vi "Get PPMS Class.vi"(8 "error in (no error)":errorcluster, 11 "instrument.PPMS":refnum<class "instrument.PPMS.lvclass">) -> (0 "error out":errorcluster, 2 "Select PPMS":T1, 3 "instrument.PPMS out":refnum<class "instrument.PPMS.lvclass">)   [LabVIEW 2019, in "PPMS.lvlib"]
uses:
  PPMS.lvlib
  Select PPMS--Enum.ctl
  instrument.PPMS/instrument.PPMS.lvclass
  instrument.PPMS1/instrument.PPMS1.lvclass
  C:/Users/patrick/Documents/GitHub/levylabpitt/PPMS-Monitor-and-Control/lvsrc/instrument.PPMS/instrument.PPMS.lvclass
  instrument.PPMS2/instrument.PPMS2.lvclass
  instrument.PPMS3/instrument.PPMS3.lvclass
  instrument.OptiCool/instrument.OptiCool.lvclass
  instrument.PPMS-W-1/instrument.PPMS-W-1.lvclass
  instrument.PPMS/instrument.PPMS.lvclass/instrument.PPMS.ctl
  C:/Program Files (x86)/National Instruments/LabVIEW 2019/user.lib/LevyLab/Instrument Framework/Instrument Types/Cryostat/Instrument.Cryostat.lvclass
  C:/Program Files (x86)/National Instruments/LabVIEW 2019/user.lib/LevyLab/Instrument Framework/Instrument/Instrument.lvclass
  C:/Program Files (x86)/National Instruments/LabVIEW 2019/vi.lib/JKI/JKI SMO/SMO/SMO.lvclass
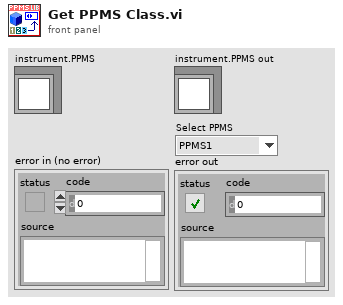
[diagram p1: front panel]
types:
  T1 = typedef "PPMS.lvlib/Select PPMS--Enum.ctl" = enum16{"PPMS1", "PPMS2", "PPMS3", "OptiCool", "PPMS-W-1", "Simulate PPMS", "Simulate DynaCool", "Simulate OptiCool"}
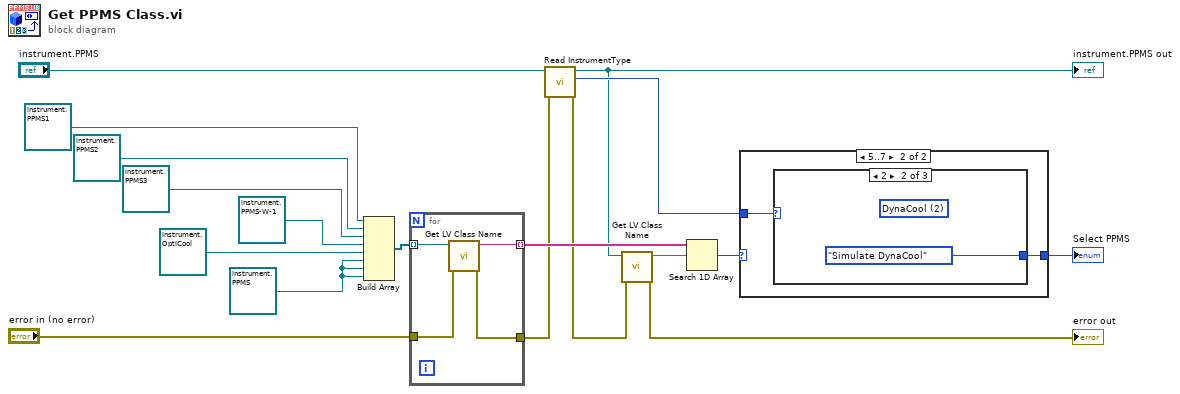
[diagram p0: block diagram]
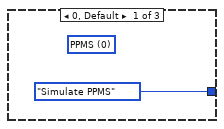
[diagram p3: hidden frame]
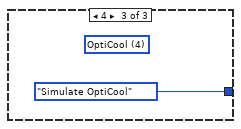
[diagram p4: hidden frame]
diagram:
  w1 = refnum<class "instrument.PPMS.lvclass"> refnum ("instrument.PPMS.lvclass")
  n1 = Build Array(refnum<class "instrument.PPMS1.lvclass"> refnum ("instrument.PPMS1.lvclass"), refnum<class "instrument.PPMS2.lvclass"> refnum ("instrument.PPMS2.lvclass"), refnum<class "instrument.PPMS3.lvclass"> refnum ("instrument.PPMS3.lvclass"), refnum<class "instrument.PPMS-W-1.lvclass"> refnum ("instrument.PPMS-W-1.lvclass"), refnum<class "instrument.OptiCool.lvclass"> refnum ("instrument.OptiCool.lvclass"), w1, w1, w1) -> (w15:refnum<class "instrument.PPMS.lvclass">[])
  n2 = for {
    tunnel: [w22] -> w14 mode=indexing
    tunnel: w15 -> [w21] mode=indexing
    tunnel: [w20] -> w6
    tunnel: "error in (no error)" -> [w19]
    n3 = call <vilib>:"Get LV Class Name.vi"("error in (no error)"=w19, "object"=w21) -> ("error out"=w20:errorcluster, "class name"=w22:string)  [unwired: 8 in]
  }
  n4 = call "Read InstrumentType.vi"("error in (no error)"=w6, "instrument.PPMS in"="instrument.PPMS") -> ("error out"=w5:errorcluster, "InstrumentType"=w7:i32, "instrument.PPMS out"=w3:refnum<class "instrument.PPMS.lvclass">)  [unwired: 7 in]
  "instrument.PPMS out" <- w3
  n5 = call <vilib>:"Get LV Class Name.vi"("error in (no error)"=w5, "object"=w3) -> ("error out"=→"error out":errorcluster, "class name"=w13:string)  [unwired: 8 in]
  n6 = Search 1D Array(1D array=w14, element=w13) -> (index of element=w9:i32)  [unwired: 1 in]
  n7 = case shown="5..7" w9 {
    selector: w9 -> [w23 _]
    tunnel: [w23 w24] -> w8
    tunnel: w7 -> [_ w25]
    frame Default {
    }
    frame 5..7 {
      n8 = case shown="2" w25 {
        tunnel: [Select_PPMS--Enum."Simulate PPMS" ("Select PPMS") Select_PPMS--Enum."Simulate DynaCool" ("Select PPMS") Select_PPMS--Enum."Simulate OptiCool" ("Select PPMS")] -> w24
        frame 0, Default {
          (unwired) 0 items=["PPMS", "VersaLab", "DynaCool", "SVSM", "OptiCool"] ("InstrumentType")
        }
        frame 2 {
          (unwired) 2 items=["PPMS", "VersaLab", "DynaCool", "SVSM", "OptiCool"] ("InstrumentType")
        }
        frame 4 {
          (unwired) 4 items=["PPMS", "VersaLab", "DynaCool", "SVSM", "OptiCool"] ("InstrumentType")
        }
      }
    }
  }
  "Select PPMS" <- w8
